vi "tipclean.vi"(8 "error in (no error)":errorcluster, 11 "Input":string="34,45,89") -> (0 "error out":errorcluster, 3 "Output":string)   [LabVIEW 2014]
uses:
  <userlib>/Nanonis Prog Interface V5/Nanonis Prog Interface.lvlib
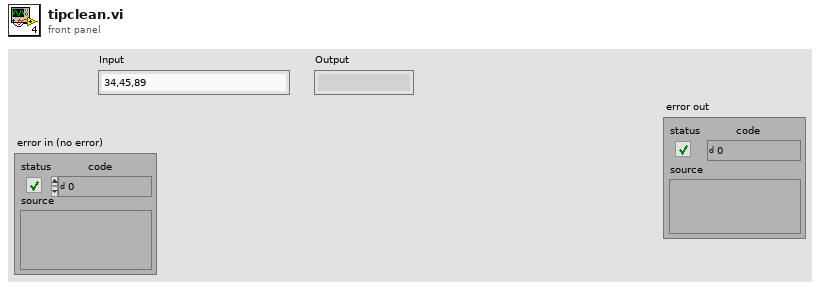
[diagram p1: front panel]
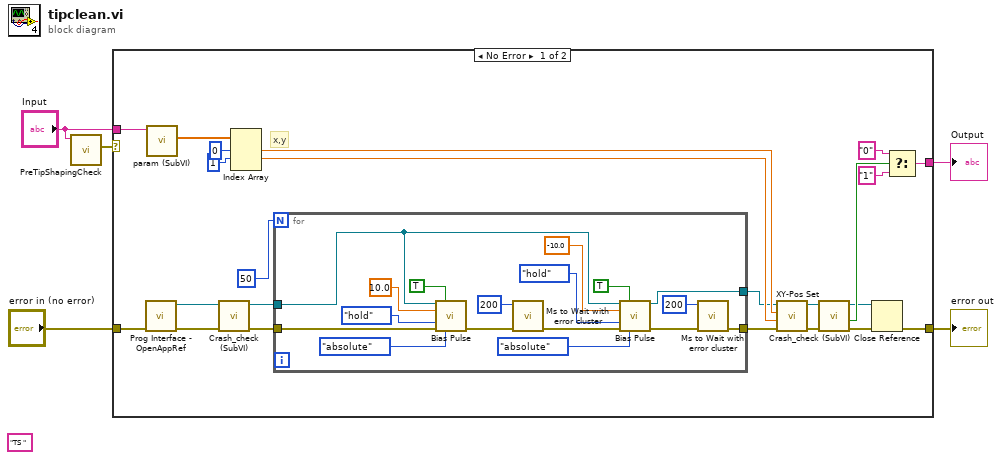
[diagram p0: block diagram]
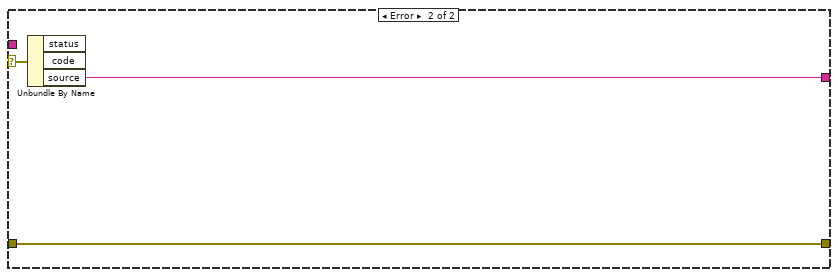
[diagram p2: hidden frame]
diagram:
  (unwired) "TS " ("string")
  n1 = call "PreTipShapingCheck.vi"("Input"="Input") -> ("Error"=w2:errorcluster)  [unwired: 8 in, 2 out]
  n2 = case shown="No Error" w2 {
    selector: w2 -> [_ w48]
    tunnel: [w9 w47] -> w5
    tunnel: "error in (no error)" -> [w27 w46]
    tunnel: "Input" -> [w22 _]
    tunnel: [w6 w46] -> w1
    frame No Error {
      # "x,y"
      n3 = call <userlib>:"Prog Interface - OpenAppRef.vi"("Error in (no error)"=w27) -> ("Error out"=w20:errorcluster, "Application reference"=w21:refnum<vi>)  [unwired: 5 in]
      n4 = call <userlib>:"param (SubVI).vi"("Input"=w22) -> ("parm"=w28:dbl[])  [unwired: 8 in, 2 out]
      n5 = call "Crash_check (SubVI).vi"("error in (no error)"=w20, "Application in"=w21) -> ("error out"=w19:errorcluster, "Application out"=w18:refnum<vi>)  [unwired: 7 in, 1 out]
      n6 = Index Array(array=w28, index #1=0 ("index"), index #2=1 ("index")) -> (element #1=w26:dbl, element #2=w25:dbl)  [unwired: 1 in, 1 out]
      n7 = for {
        N: 50 -> [_]
        tunnel: w19 -> [w45]
        tunnel: w18 -> [w35]
        tunnel: [w30] -> w16
        tunnel: [w29] -> w15
        n8 = call <userlib>:"Bias Pulse.vi"("Application ref in"=w35, "Wait until done (T)"=TRUE, "Pulse bias (V) (1)"=10.0, "Z-Controller (no change)"=enum16{"no change", "hold", "don't hold"}."hold", "Error in (no error)"=w45, "Pulse abs/rel (no change)"=enum16{"no change", "relative", "absolute"}."absolute") -> ("Error out"=w44:errorcluster)  [unwired: 8 in, 1 out]
        n9 = call <userlib>:"Ms to Wait with error cluster.vi"("error in (no error)"=w44, "milliseconds to wait"=u32 200) -> ("error out"=w34:errorcluster)  [unwired: 4 in, 1 out]
        n10 = call <userlib>:"Bias Pulse.vi"("Application ref in"=w35, "Wait until done (T)"=TRUE, "Pulse bias (V) (1)"=-10.0, "Z-Controller (no change)"=enum16{"no change", "hold", "don't hold"}."hold", "Error in (no error)"=w34, "Pulse abs/rel (no change)"=enum16{"no change", "relative", "absolute"}."absolute") -> ("Application ref out"=w30:refnum<vi>, "Error out"=w33:errorcluster)  [unwired: 8 in]
        n11 = call <userlib>:"Ms to Wait with error cluster.vi"("error in (no error)"=w33, "milliseconds to wait"=u32 200) -> ("error out"=w29:errorcluster)  [unwired: 4 in, 1 out]
      }
      n12 = call <userlib>:"XY-Pos Set.vi"("error in (no error)"=w15, "Y (m)"=w25, "X (m)"=w26, "Application ref in"=w16) -> ("error out"=w13:errorcluster, "Application ref out"=w14:refnum<vi>)  [unwired: 4 in]
      n13 = call "Crash_check (SubVI).vi"("error in (no error)"=w13, "Application in"=w14) -> ("error out"=w7:errorcluster, "x > y?"=w11:bool, "Application out"=w8:refnum<vi>)  [unwired: 7 in]
      n14 = Close Reference(reference=w8, error in (no error)=w7) -> (error out=w6:errorcluster)
      n15 = Select(t="0", s=w11, f="1") -> (s? t:f=w9:string)
    }
    frame Error {
      n16 = Unbundle By Name(w48) -> ("source"=w47:string)  [unwired: 2 out]
    }
  }
  "Output" <- w5
  "error out" <- w1
